vi "Wire Encode Tag.vi"(7 "Field Number":i32, 10 "Wire Type":T1, 11 "Buffer in":u8[](array[numeric]) format="%.0x") -> (3 "Buffer":u8[](array[numeric]) format="%.0x")   [LabVIEW 2020, in "LV-Proto.lvlib"]
uses:
  LV-Proto.lvlib
  Wire Type.ctl
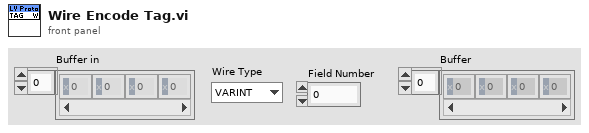
[diagram p1: front panel]
types:
  T1 = typedef "LV-Proto.lvlib/Wire Type.ctl" = enum8{"VARINT", "I64", "LEN", "SGROUP (Deprecated)", "EGROUP (Deprecated)", "I32"}
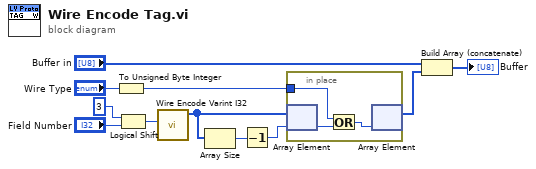
[diagram p0: block diagram]
diagram:
  n1 = To Unsigned Byte Integer(number="Wire Type") -> (unsigned 8bit integer=w4:u8)
  n2 = Logical Shift(y=i16 3, x="Field Number") -> (x << y=w9:i32)
  n3 = call "Wire Encode Varint I32.vi"("I32"=w9) -> ("Buffer"=w6:u8[])  [unwired: 10 in]
  n4 = Array Size(array=w6) -> (size(s)=w7:i32)
  n5 = Decrement(x=w7) -> (x-1=w5:i32)
  n6 = in-place {
    in-place-border: w4 -> [w13]
    n7 = in-place-array #1(w6, w5) -> (w14:u8)
    n8 = Or(x=w13, y=w14) -> (x .or. y?=w12:u8)
    n9 = in-place-array #1(w12) -> (w2:u8[])  [unwired: 1 out]
  }
  n10 = Build Array (concatenate)("Buffer in", w2) -> (→"Buffer":u8[])
